vi "Interface.vi"(8 "error in (no error)":errorcluster, 11 "Node Ptr":T1 format="%.0x") -> (0 "error out":errorcluster)   [LabVIEW 2017, in "NI-XNET Monitor System Explorer.lvlib"]
uses:
  NI-XNET Monitor System Explorer.lvlib
  <vilib>/NI Veristand/Custom Device API/Custom Device Item Ref.ctl
  <vilib>/NI Veristand/Custom Device API/Custom Device API.lvlib
panel:
  in  "Header":cluster{"Section Name":string}={"Section Name"=" Section"}
  in  "Description":string
  in  "Name":string
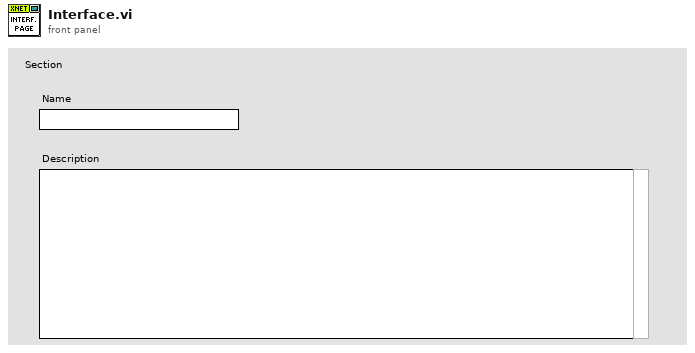
[diagram p1: front panel]
types:
  T1 = typedef "Custom Device API.lvlib/Custom Device Item Ref.ctl" = u64
  T2 = typedef "Custom Device API.lvlib/Custom Device Item Info.ctl" = cluster{"Name":string, "Is Channel":bool, "GUID":string, "Is Waveform":bool}
  T3 = typedef "Custom Device API.lvlib/Custom Device Commands.ctl" = enum16{"Default", "Item renamed", "Shutdown", "Dynamic button pressed"}
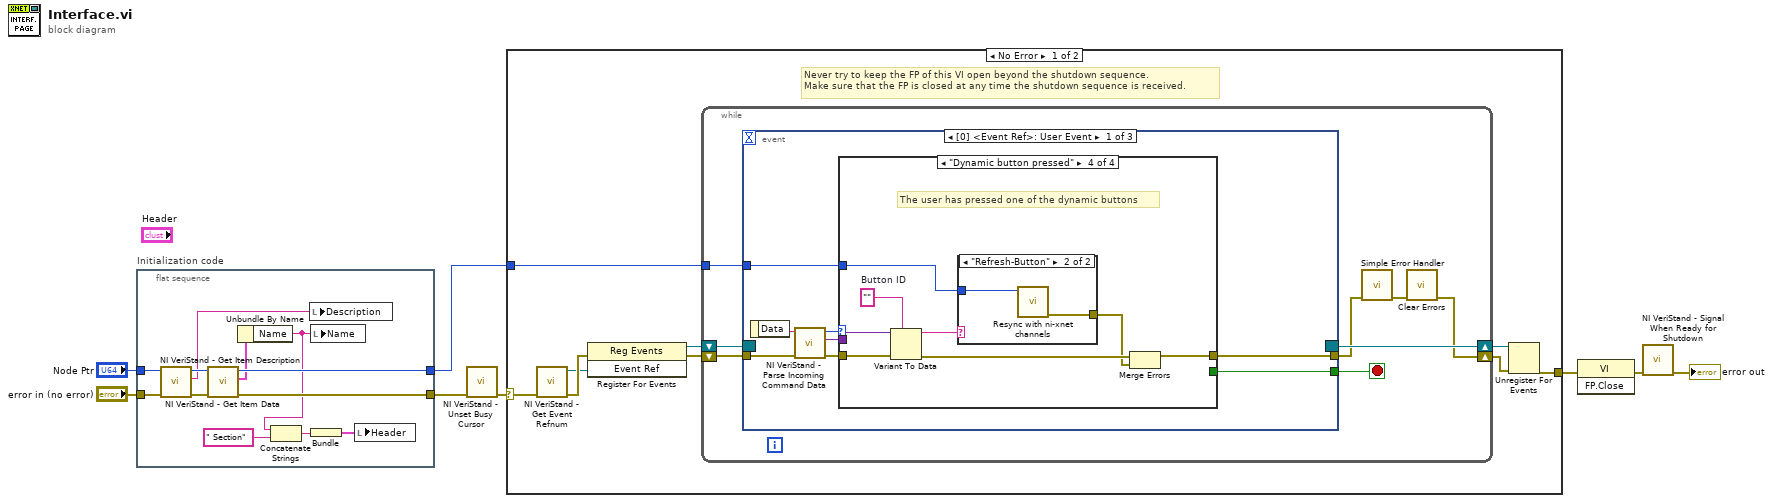
[diagram p0: block diagram]
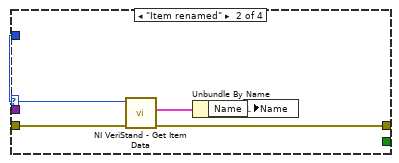
[diagram p3: hidden frame]
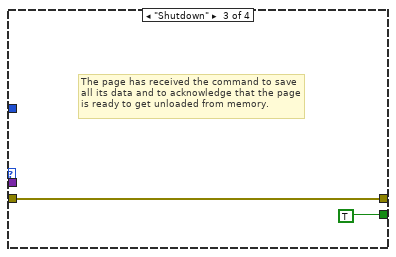
[diagram p4: hidden frame]
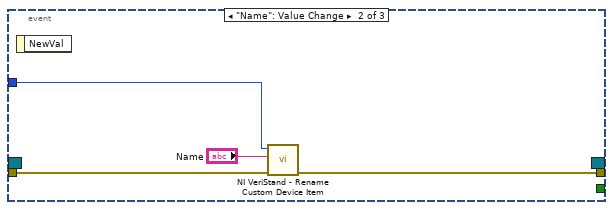
[diagram p6: hidden frame]
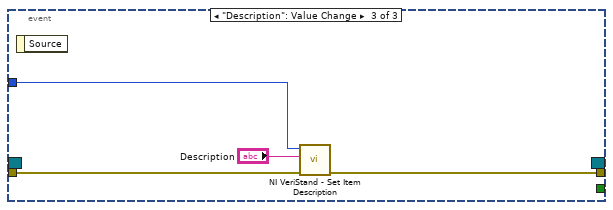
[diagram p7: hidden frame]
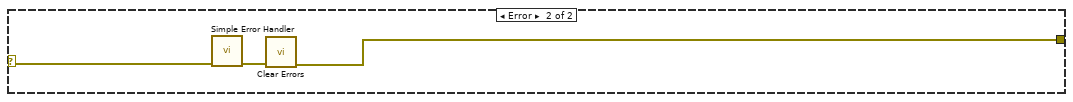
[diagram p8: hidden frame]
diagram:
  n1 = flat-sequence "Initialization code" {
    tunnel: "error in (no error)" -> [w18]
    tunnel: "Node Ptr" -> [w17]
    tunnel: [w13] -> w4
    tunnel: [w20] -> w1
    frame #0 {
      n2 = call <vilib>:"NI VeriStand - Get Item Description.vi"("error in (no error)"=w18, "Item Ref in"=w17) -> ("error out"=w15:errorcluster, "Description"=w16:string, "Item Ref out"=w19:T1)  [unwired: 7 out]
      n3 = call <vilib>:"NI VeriStand - Get Item Data.vi"("error in (no error)"=w15, "Item Ref in"=w19) -> ("error out"=w13:errorcluster, "Item Info"=w14:T2, "Item Ref out"=w20:T1)  [unwired: 7 out]
      n4 = Unbundle By Name(w14) -> ("Name"=w10:string)
      n5 = Concatenate Strings(w10, " Section" ("Section Name")) -> (w12:string)
      n6 = local write "Description"(w16) -> ()
      n7 = local write "Name"(w10) -> ()
      n8 = Bundle(w12) -> (w11:cluster{string})  [unwired: 1 in]
      n9 = local write "Header"(w11) -> ()
    }
  }
  n10 = call <vilib>:"NI VeriStand - Unset Busy Cursor.vi"("error in (no error)"=w4) -> ("error out"=w3:errorcluster)  [unwired: 10 out]
  n11 = case shown="No Error" w3 {
    selector: w3 -> [w21 w74]
    tunnel: [w26 w72] -> w8
    tunnel: w1 -> [w22 _]
    frame No Error {
      # "Never try to keep the FP of this VI open beyond the shutdown sequence.\nMake sure that the FP is closed at any time the shutdown sequence is received."
      n12 = call <vilib>:"NI VeriStand - Get Event Refnum.vi"("error in (no error)"=w21) -> ("error out"=w29:errorcluster, "Event Ref"=w25:refnum<user-event>)  [unwired: 9 out]
      n13 = register-events(error in=w29, w25) -> (reference out=w23:refnum<event-registration>, error out=w24:errorcluster)  [unwired: 1 in]
      n14 = while {
        tunnel: w22 -> [w33]
        shift-right: [w30] -> w27
        shift-left: w24 -> [w36]
        shift-right: [w37] -> w28
        shift-left: w23 -> [w35]
        stop <- w34 stop-if-true
        n15 = event shown="[0] <Event Ref>: User Event" {
          selector: w35 -> [_ _ _]
          dyn-events: [_ _ _] -> w37
          timeout: _ -> [_ _ _]
          tunnel: w36 -> [w45 w67 w70]
          tunnel: [w41 _ _] -> w34
          tunnel: [w40 w66 w69] -> w32
          tunnel: w33 -> [w39 w65 w71]
          event User Event {
            n16 = event-data() -> ("Data"=w44:string)  [unwired: 1 out]
            n17 = call <vilib>:"NI VeriStand - Parse Incoming Command Data.vi"("error in (no error)"=w45, "Incoming data"=w44) -> ("error out"=w43:errorcluster, "Outgoing data"=w38:variant, "Action"=w42:T3)  [unwired: 7 out]
            n18 = case shown="\"Dynamic button pressed\"" w42 {
              tunnel: w43 -> [w46 w51 w52 w61]
              tunnel: [_ _ TRUE _] -> w41
              tunnel: [w46 w48 w52 w55] -> w40
              tunnel: w39 -> [_ w50 _ w57]
              tunnel: w38 -> [_ _ _ w60]
              frame "Default", Default {
              }
              frame "Item renamed" {
                n19 = call <vilib>:"NI VeriStand - Get Item Data.vi"("error in (no error)"=w51, "Item Ref in"=w50) -> ("error out"=w48:errorcluster, "Item Info"=w49:T2)  [unwired: 8 out]
                n20 = Unbundle By Name(w49) -> ("Name"=w47:string)
                n21 = local write "Name"(w47) -> ()
              }
              frame "Shutdown" {
                # "The page has received the command to save all its data and to acknowledge that the page is ready to get unloaded from memory."
              }
              frame "Dynamic button pressed" {
                w59 = ""  # Button ID
                # "The user has pressed one of the dynamic buttons"
                n22 = Variant To Data(error in=w61, type=w59, Variant=w60) -> (data=w56:string, error out=w58:errorcluster)
                n23 = case shown="\"Refresh-Button\"" w56 {
                  tunnel: w57 -> [_ w63]
                  tunnel: [_ w62] -> w54
                  frame Default {
                  }
                  frame "Refresh-Button" {
                    n24 = call "Resync with ni-xnet channels.vi"("Device Item Ref in in"=w63) -> ("Error Out"=w62:errorcluster)  [unwired: 9 in, 1 out]
                  }
                }
                n25 = Merge Errors(w58, w54) -> (w55:errorcluster)
              }
            }
          }
          event "Name": Value Change {
            n26 = event-data() -> ()  [unwired: 2 out]
            n27 = call <vilib>:"NI VeriStand - Rename Custom Device Item.vi"("error in (no error)"=w67, "New Name"="Name", "Item Ref in"=w65) -> ("error out"=w66:errorcluster)  [unwired: 1 in, 7 out]
          }
          event "Description": Value Change {
            n28 = event-data() -> ()  [unwired: 2 out]
            n29 = call <vilib>:"NI VeriStand - Set Item Description.vi"("error in (no error)"=w70, "Description"="Description", "Item Ref in"=w71) -> ("error out"=w69:errorcluster)  [unwired: 8 out]
          }
        }
        n30 = call <vilib>:"Simple Error Handler.vi"("error in (no error)"=w32) -> ("error out"=w31:errorcluster)  [unwired: 1 in, 7 out]
        n31 = call <vilib>:"Clear Errors.vi"("error in (no error)"=w31) -> ("error out"=w30:errorcluster)  [unwired: 1 in, 5 out]
      }
      n32 = Unregister For Events(event registration refnum=w28, error in=w27) -> (error out=w26:errorcluster)
    }
    frame Error {
      n33 = call <vilib>:"Simple Error Handler.vi"("error in (no error)"=w74) -> ("error out"=w73:errorcluster)  [unwired: 1 in, 7 out]
      n34 = call <vilib>:"Clear Errors.vi"("error in (no error)"=w73) -> ("error out"=w72:errorcluster)  [unwired: 1 in, 5 out]
    }
  }
  n35 = invoke class="VI" method="FP.Close"(error in=w8) -> (error out=w7:errorcluster)  [unwired: 2 in, 2 out]
  n36 = call <vilib>:"NI VeriStand - Signal When Ready for Shutdown.vi"("error in (no error)"=w7) -> ("error out"=→"error out":errorcluster)  [unwired: 10 out]
